vi "Get Summary.vi"(8 "error in (no error)":errorcluster, 10 "Item":string, 11 "Result Model In":refnum<class "Result Model.lvclass">) -> (0 "error out":errorcluster, 2 "Summary":string, 3 "Result Model Out":refnum<class "Result Model.lvclass">)   [LabVIEW 2020, in "Result Model.lvclass"]
uses:
  Result Model.lvclass
  Result/Status.ctl
  Result Model.lvclass/Result Model.ctl
  Result/Result.lvlib
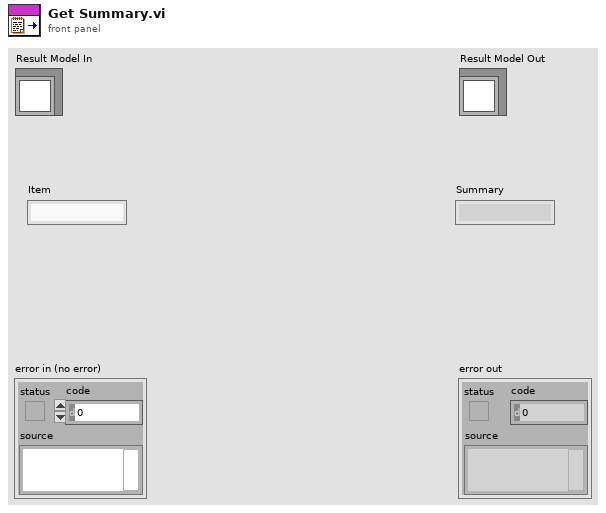
[diagram p1: front panel]
types:
  T1 = typedef "Result.lvlib/Status.ctl" = enum16{"", "Passed", "Failed", "Error", "Skipped", "Setup Error", "Broken", "Teardown Error"}
  T2 = map{cluster{"Test Case":string, "Status":T1}, i32}
  T3 = typedef "Result Model.lvclass/Test Model.ctl" = cluster{"Status":T1, "Summary":string}
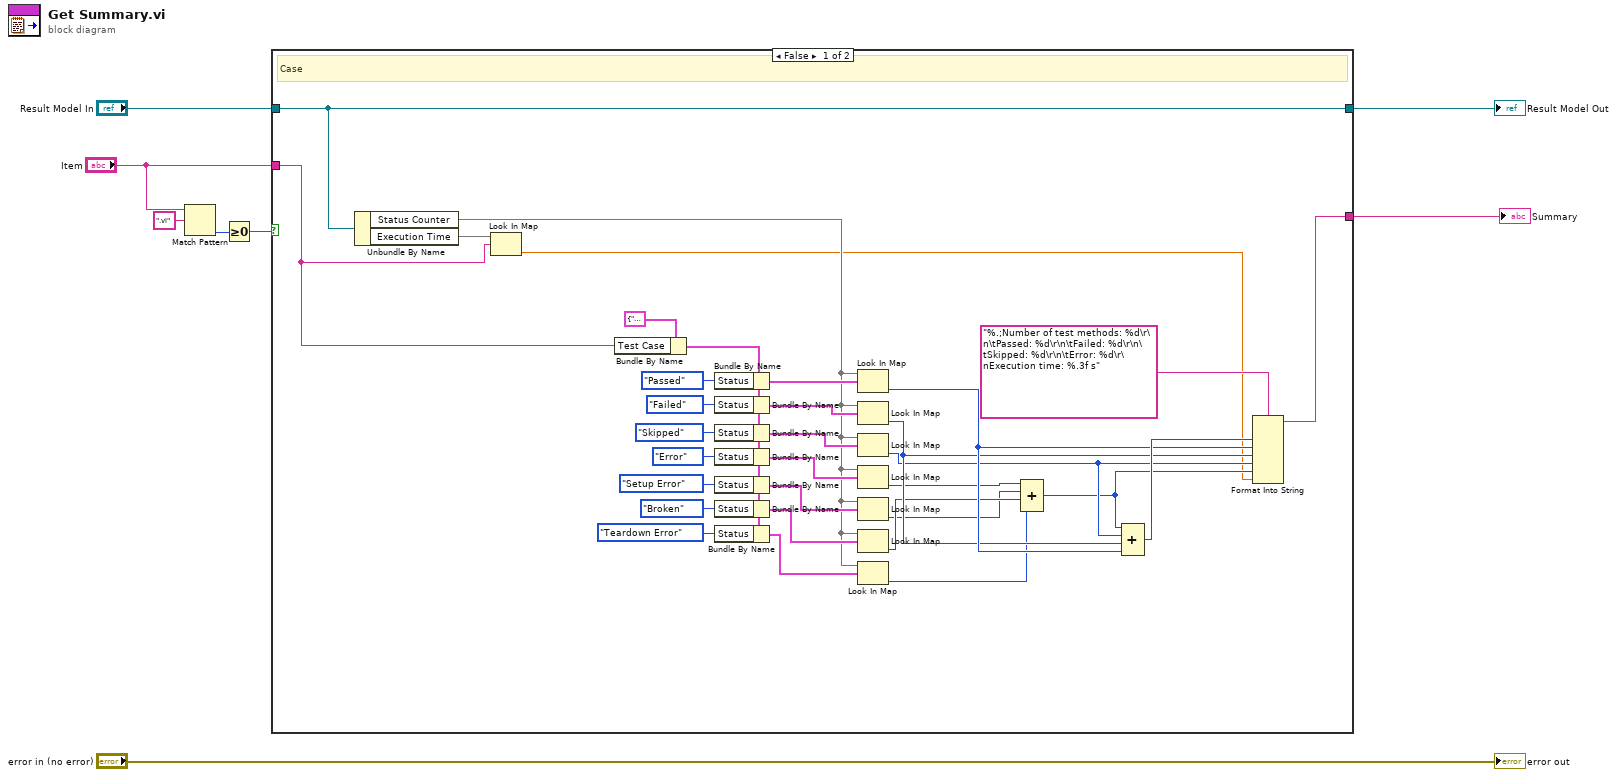
[diagram p0: block diagram]
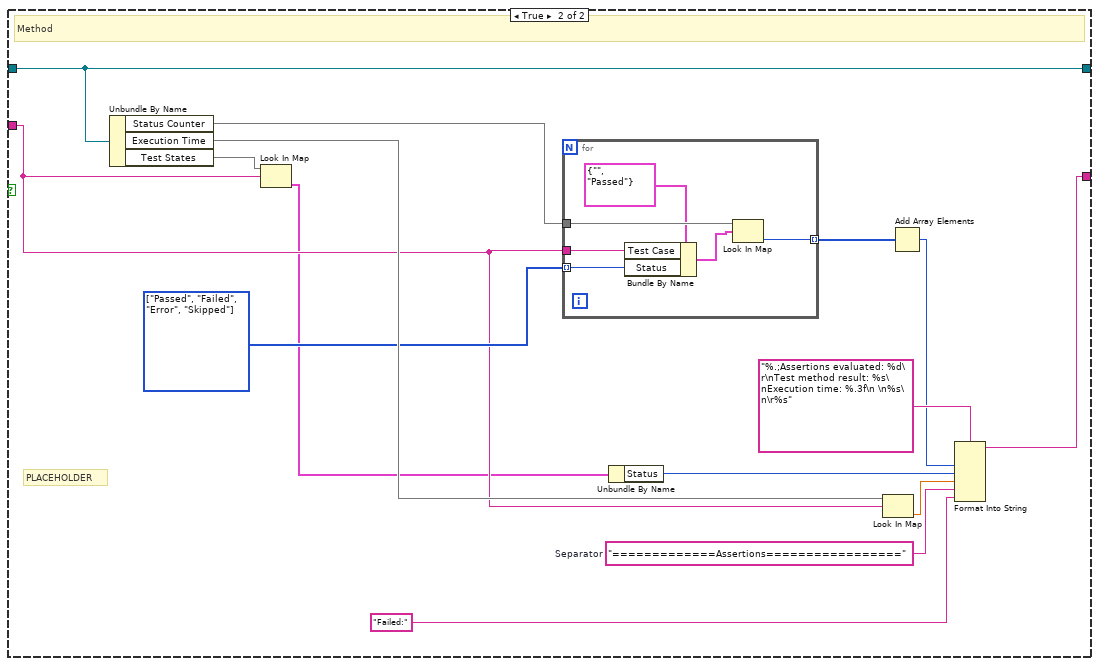
[diagram p2: hidden frame]
diagram:
  n1 = Match Pattern(string="Item", regular expression=".vi") -> (offset past match=w6:i32)  [unwired: 1 in, 3 out]
  n2 = Greater Or Equal To 0?(x=w6) -> (x >= 0?=w5:bool)
  n3 = case shown="False" w5 {
    tunnel: "Result Model In" -> [w40 w48]
    tunnel: "Item" -> [w10 w43]
    tunnel: [w12 w46] -> w2
    tunnel: [w40 w48] -> w1
    frame False {
      # "Case"
      n4 = Unbundle By Name(w40) -> ("Status Counter"=w15:T2, "Execution Time"=w11:map{string, dbl})
      n5 = Look In Map(map=w11, key=w10) -> (value=w9:dbl)  [unwired: 1 in, 1 out]
      n6 = Bundle By Name(cluster=cluster{"Test Case":string, "Status":T1} {"Test Case"="", "Status"=enum."Passed"} ("key"), "Test Case"=w10) -> (w13:cluster{"Test Case":string, "Status":T1})
      n7 = Bundle By Name(cluster=w13, "Status"=Status."Passed") -> (w18:cluster{"Test Case":string, "Status":T1})
      n8 = Bundle By Name(cluster=w13, "Status"=Status."Failed") -> (w20:cluster{"Test Case":string, "Status":T1})
      n9 = Bundle By Name(cluster=w13, "Status"=Status."Skipped") -> (w22:cluster{"Test Case":string, "Status":T1})
      n10 = Bundle By Name(cluster=w13, "Status"=Status."Error") -> (w23:cluster{"Test Case":string, "Status":T1})
      n11 = Bundle By Name(cluster=w13, "Status"=Status."Setup Error") -> (w29:cluster{"Test Case":string, "Status":T1})
      n12 = Bundle By Name(cluster=w13, "Status"=Status."Broken") -> (w30:cluster{"Test Case":string, "Status":T1})
      n13 = Bundle By Name(cluster=w13, "Status"=Status."Teardown Error") -> (w39:cluster{"Test Case":string, "Status":T1})
      n14 = Look In Map(map=w15, key=w18) -> (value=w37:i32)  [unwired: 1 in, 1 out]
      n15 = Look In Map(map=w15, key=w20) -> (value=w36:i32)  [unwired: 1 in, 1 out]
      n16 = Look In Map(map=w15, key=w22) -> (value=w35:i32)  [unwired: 1 in, 1 out]
      n17 = Look In Map(map=w15, key=w23) -> (value=w24:i32)  [unwired: 1 in, 1 out]
      n18 = Look In Map(map=w15, key=w29) -> (value=w31:i32)  [unwired: 1 in, 1 out]
      n19 = Look In Map(map=w15, key=w30) -> (value=w32:i32)  [unwired: 1 in, 1 out]
      n20 = Look In Map(map=w15, key=w39) -> (value=w33:i32)  [unwired: 1 in, 1 out]
      n21 = Compound Arithmetic op=ADD(w24, w31, w32, w33) -> (w34:i32)
      n22 = Compound Arithmetic op=ADD(w34, w35, w36, w37) -> (w38:i32)
      n23 = Format Into String(format string="%.;Number of test methods: %d\r\n\tPassed: %d\r\n\tFailed: %d\r\n\tSkipped: %d\r\n\tError: %d\r\nExecution time: %.3f s", w38, w37, w36, w35, w34, w9) -> (resulting string=w12:string)  [unwired: 2 in, 1 out]
    }
    frame True {
      w47 = T1[] [enum."Passed", enum."Failed", enum."Error", enum."Skipped"] items=["", "Passed", "Failed", "Error", "Skipped", "Setup Error", "Broken", "Teardown Error"] ("Array")
      w54 = "=============Assertions================="  # Separator
      # "PLACEHOLDER"
      # "Method"
      n24 = Unbundle By Name(w48) -> ("Status Counter"=w53:T2, "Execution Time"=w50:map{string, dbl}, "Test States"=w44:map{string, T3})
      n25 = Look In Map(map=w44, key=w43) -> (value=w42:T3)  [unwired: 1 in, 1 out]
      n26 = for {
        tunnel: w53 -> [w61]
        tunnel: w43 -> [w58]
        tunnel: w47 -> [w57] mode=indexing
        tunnel: [w56] -> w52 mode=indexing
        n27 = Bundle By Name(cluster=cluster{"Test Case":string, "Status":T1} {"Test Case"="", "Status"=enum."Passed"} ("key"), "Test Case"=w58, "Status"=w57) -> (w59:cluster{"Test Case":string, "Status":T1})
        n28 = Look In Map(map=w61, key=w59) -> (value=w56:i32)  [unwired: 1 in, 1 out]
      }
      n29 = Unbundle By Name(w42) -> ("Status"=w41:T1)
      n30 = Look In Map(map=w50, key=w43) -> (value=w49:dbl)  [unwired: 1 in, 1 out]
      n31 = Add Array Elements(numeric array=w52) -> (sum=w51:i32)
      n32 = Format Into String(format string="%.;Assertions evaluated: %d\r\nTest method result: %s\nExecution time: %.3f\n \n%s\n\r%s", w51, w41, w49, w54, "Failed:" ("input 5")) -> (resulting string=w46:string)  [unwired: 2 in, 1 out]
    }
  }
  "Result Model Out" <- w1
  "Summary" <- w2
  "error out" <- "error in (no error)"
